vi "lvGraphProfile.vi"(0 "pathToJson":path=path "C:/Users/stefan/Documents/GitHub/TVAC/head/Labview2017/TVAC_GUI/TestScripts/graphTest.json", 5 "error in (no error)":errorcluster, 7 "pathToJson 2":path=path "C:/Users/stefan/Documents/GitHub/TVAC/head/Labview2017/TVAC_GUI/TestScripts/graphTest.json", 9 "Path to Python.exe":path=path "C:/ProgramData/Anaconda3/python.exe", 11 "RunCount":dbl) -> (4 "graphCluster":T1, 8 "Raw Python String Output":string, 15 "error out":errorcluster)   [LabVIEW 2017]
uses:
  <vilib>/Utility/error.llb/DialogType.ctl
panel:
  out "Standard Error":string
  out "Return Code":i32
  # "1. Inputs - Set before running VI"
  # "2. Outputs"
  # "3. Errors - Both Standard and LabVIEW"
  # "A + B ="
  # "This VI sends inputs to a simple Python script, and returns its output.\n\nSee block diagram for code and comments"
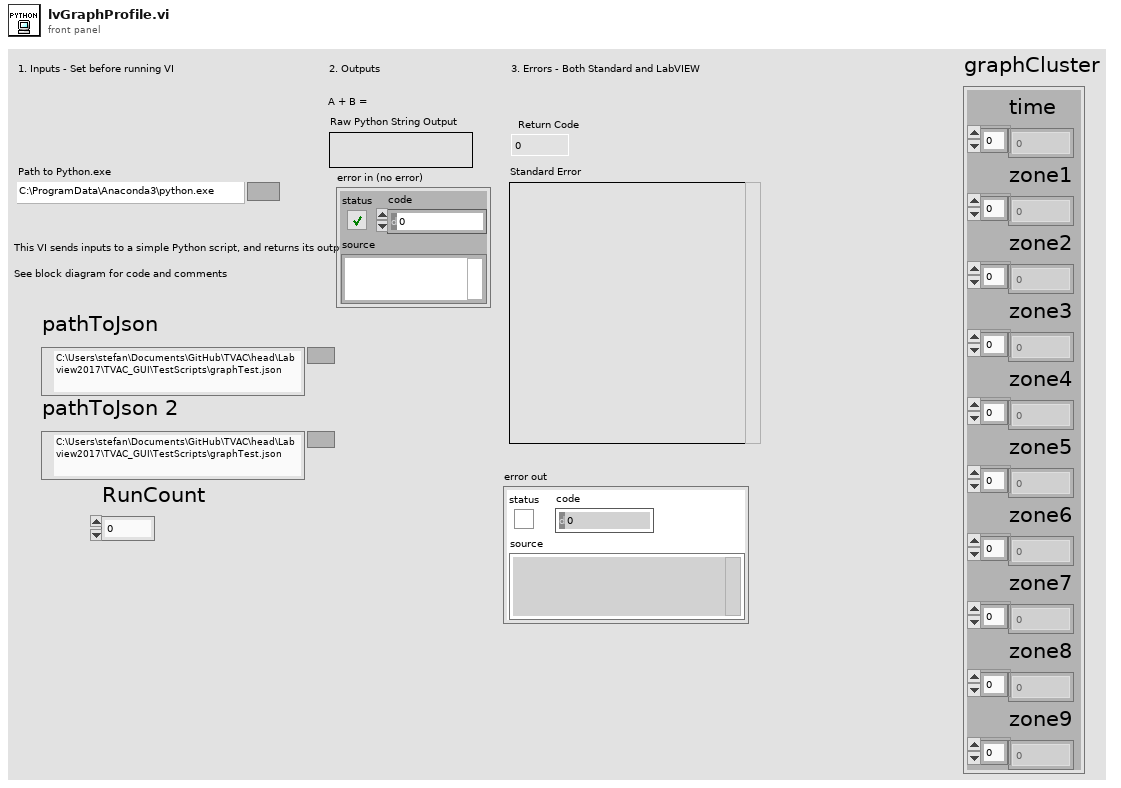
[diagram p1: front panel]
types:
  T1 = cluster{"time":dbl[], "zone1":dbl[], "zone2":dbl[], "zone3":dbl[], "zone4":dbl[], "zone5":dbl[], "zone6":dbl[], "zone7":dbl[], "zone8":dbl[], "zone9":dbl[]}
  T2 = typedef "DialogType.ctl" = u16
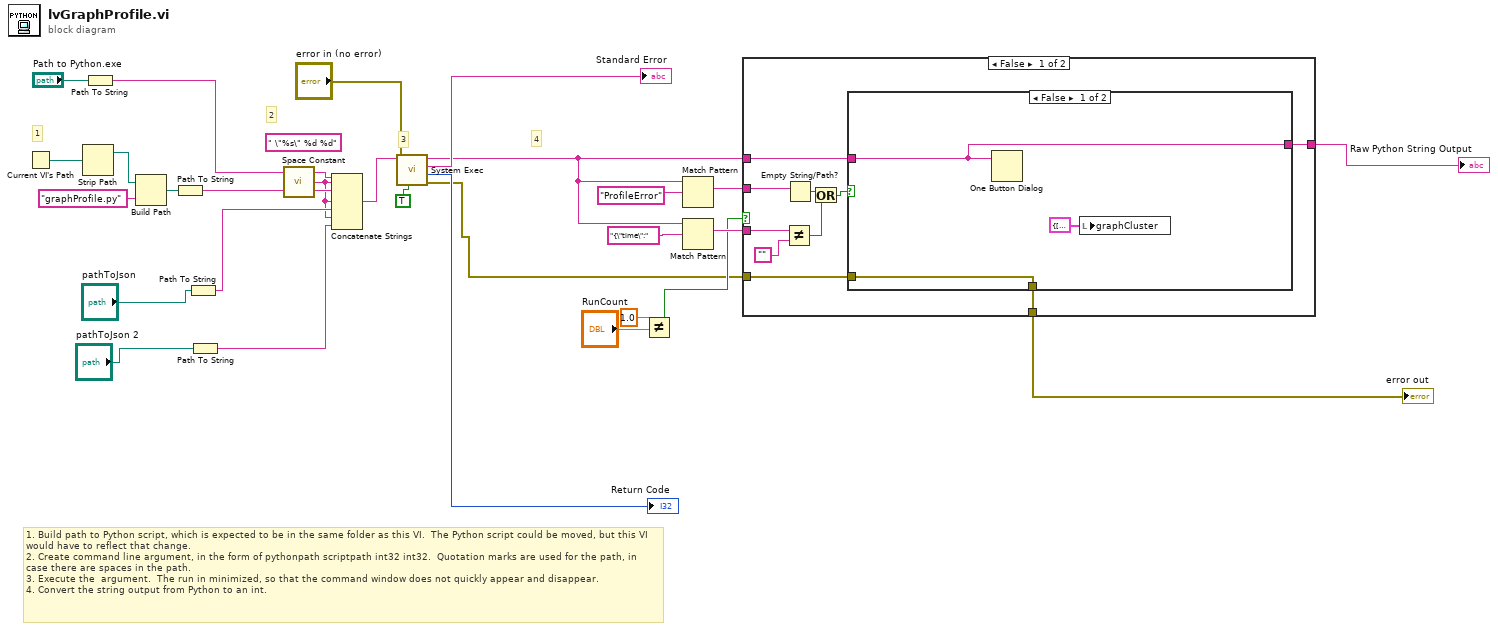
[diagram p0: block diagram]
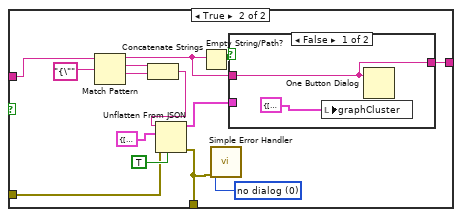
[diagram p2: hidden frame]
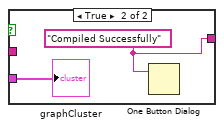
[diagram p3: hidden frame]
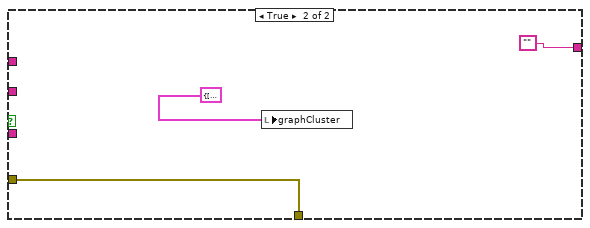
[diagram p4: hidden frame]
diagram:
  (unwired) " \"%s\" %d %d" ("format string")
  # "1. Build path to Python script, which is expected to be in the same folder as this VI.  The Python script could be moved, but this VI would have to reflect that change.\n2. Create command line argument, in the form of pythonpath scriptpath int32 int32.  Quotation marks are used for the path, in case there are spaces in the path.\n3. Execute the  argument.  The run in minimized, so that the command window does not quickly appear and disappear.\n4. Convert the string output from Python to an int."
  # "4"
  # "3"
  # "2"
  # "1"
  n1 = Current VI's Path() -> (path=w23:path)
  n2 = Strip Path(path=w23) -> (stripped path=w21:path)  [unwired: 1 out]
  n3 = Path To String(path="Path to Python.exe") -> (string=w18:string)
  n4 = Build Path(base path=w21, name or relative path="graphProfile.py" ("Path to Function")) -> (appended path=w24:path)
  n5 = Path To String(path=w24) -> (string=w19:string)
  n6 = Path To String(path="pathToJson") -> (string=w16:string)
  n7 = Path To String(path="pathToJson 2") -> (string=w4:string)
  n8 = call <vilib>:"Space Constant.vi"() -> ("String"=w3:string)
  n9 = Concatenate Strings(w18, w3, w19, w3, w16, w3, w4) -> (w20:string)
  n10 = call <vilib>:"System Exec.vi"("run minimized? (F)"=TRUE, "error in (no error)"="error in (no error)", "command line"=w20) -> ("error out"=w2:errorcluster, "return code"=→"Return Code":i32, "standard error"=→"Standard Error":string, "standard output"=w11:string)  [unwired: 5 in]
  n11 = Not Equal?(x=1.0, y="RunCount") -> (x != y?=w7:bool)
  n12 = Match Pattern(string=w11, regular expression="ProfileError") -> (match substring=w13:string)  [unwired: 1 in, 3 out]
  n13 = Match Pattern(string=w11, regular expression="{\"time\":") -> (match substring=w10:string)  [unwired: 1 in, 3 out]
  n14 = case shown="False" w7 {
    tunnel: w13 -> [w38 _]
    tunnel: w11 -> [w35 _]
    tunnel: w10 -> [w32 _]
    tunnel: [w31 ""] -> w6
    tunnel: w2 -> [w30 w60]
    tunnel: [w29 w60] -> w1
    frame False {
      n15 = Not Equal?(x=w32, y="") -> (x != y?=w34:bool)
      n16 = Empty String/Path?(string/path=w38) -> (empty?=w36:bool)
      n17 = Or(x=w36, y=w34) -> (x .or. y?=w37:bool)
      n18 = case shown="False" w37 {
        tunnel: w35 -> [w41 w54]
        tunnel: [w41 w47] -> w31
        tunnel: w30 -> [w39 w44]
        tunnel: [w39 w43] -> w29
        frame False {
          n19 = One Button Dialog(message=w41) -> ()  [unwired: 1 in, 1 out]
          n20 = local write "graphCluster"(T1 {"time"=[], "zone1"=[], "zone2"=[], "zone3"=[], "zone4"=[], "zone5"=[], "zone6"=[], "zone7"=[], "zone8"=[], "zone9"=[]} ("graphCluster")) -> ()
        }
        frame True {
          w42 = T2 0 items=["no dialog", "OK message", "continue or stop message", "OK message + warnings", "continue/stop + warnings"] ("type of dialog (OK msg:1)")
          n21 = Match Pattern(string=w54, regular expression="{\"") -> (before substring=w48:string, match substring=w52:string, after substring=w51:string)  [unwired: 1 in, 1 out]
          n22 = Concatenate Strings(w52, w51) -> (w50:string)
          n23 = Unflatten From JSON(JSON string=w50, type and defaults=T1 {"time"=[], "zone1"=[], "zone2"=[], "zone3"=[], "zone4"=[], "zone5"=[], "zone6"=[], "zone7"=[], "zone8"=[], "zone9"=[]}, default null elements? (F)=TRUE, error in (no error)=w44) -> (value=w45:T1, error out=w43:errorcluster)  [unwired: 3 in]
          n24 = Empty String/Path?(string/path=w48) -> (empty?=w49:bool)
          n25 = call <vilib>:"Simple Error Handler.vi"("type of dialog (OK msg:1)"=w42, "error in (no error)"=w43) -> ()  [unwired: 3 in, 5 out]
          n26 = case shown="False" w49 {
            tunnel: w48 -> [w57 _]
            tunnel: [w57 w59] -> w47
            tunnel: w45 -> [_ w58]
            frame False {
              n27 = local write "graphCluster"(T1 {"time"=[], "zone1"=[], "zone2"=[], "zone3"=[], "zone4"=[], "zone5"=[], "zone6"=[], "zone7"=[], "zone8"=[], "zone9"=[]} ("graphCluster")) -> ()
              n28 = One Button Dialog(message=w57) -> ()  [unwired: 1 in, 1 out]
            }
            frame True {
              w59 = "Compiled Successfully" ("message")
              n29 = One Button Dialog(message=w59) -> ()  [unwired: 1 in, 1 out]
              "graphCluster" <- w58
            }
          }
        }
      }
    }
    frame True {
      n30 = local write "graphCluster"(T1 {"time"=[], "zone1"=[], "zone2"=[], "zone3"=[], "zone4"=[], "zone5"=[], "zone6"=[], "zone7"=[], "zone8"=[], "zone9"=[]}) -> ()
    }
  }
  "error out" <- w1
  "Raw Python String Output" <- w6
